vi "video.update_set_property.vi"(8 "error in":errorcluster, 11 "VideoUpdateStaging in":refnum<class "VideoUpdateStaging.lvclass">) -> (0 "error out":errorcluster, 3 "VideoUpdateStaging out":refnum<class "VideoUpdateStaging.lvclass">)   [LabVIEW 2020, in "VideoUpdateStaging.lvclass"]
doc: "Sets a property that will be included in the property set replacing the video's current properties."
uses:
  VideoUpdateStaging.lvclass
  VideoUpdateStaging.lvclass/VideoUpdateStaging.ctl
  client.lvlib
panel:
  in  "key":string
  in  "value":string
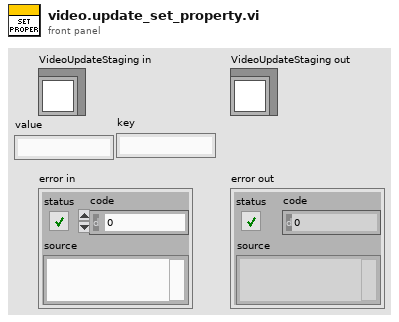
[diagram p1: front panel]
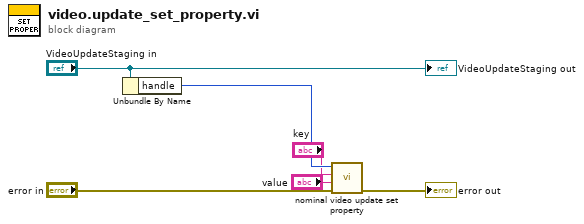
[diagram p0: block diagram]
diagram:
  n1 = Unbundle By Name("VideoUpdateStaging in") -> ("handle"=w4:i32)
  n2 = call "nominal video update set property.vi"("error in (no error)"="error in", "value"="value", "key"="key", "staging"=w4) -> ("error out"=→"error out":errorcluster)  [unwired: 6 in, 1 out]
  "VideoUpdateStaging out" <- "VideoUpdateStaging in"
